vi "DualEncoder.vi"(8 "error in (no error)":errorcluster, 11 "Reset?":bool) -> (0 "error out":errorcluster, 1 "Distance Right (in)":dbl, 2 "Distance Left (in)":dbl, 3 "Total Distance (in)":dbl, 4 "Angle (degrees)":dbl)   [LabVIEW 2012]
uses:
  Robot Global Data.vi
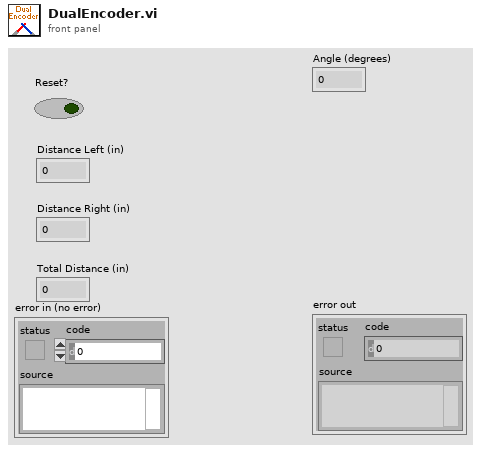
[diagram p1: front panel]
types:
  T1 = typedef "WPI_EncoderDevRef.ctl" = cluster{"DevStatus":errorcluster, "EncoderIndex":T2, "CounterIndex":T3, "DistancePerCount":dbl, "Decoding Type":T4}
  T2 = typedef "FPGA_EncoderIdx.ctl" = enum8{"Enc 0", "Enc 1", "Enc 2", "Enc 3", "Invalid"}
  T3 = typedef "FPGA_CounterCtrSystemIndex.ctl" = enum8{"Ctr 0", "Ctr 1", "Ctr 2", "Ctr 3", "Ctr 4", "Ctr 5", "Ctr 6", "Ctr 7", "Invalid"}
  T4 = typedef "WPI_EncoderType.ctl" = enum16{"1x", "2x", "4x"}
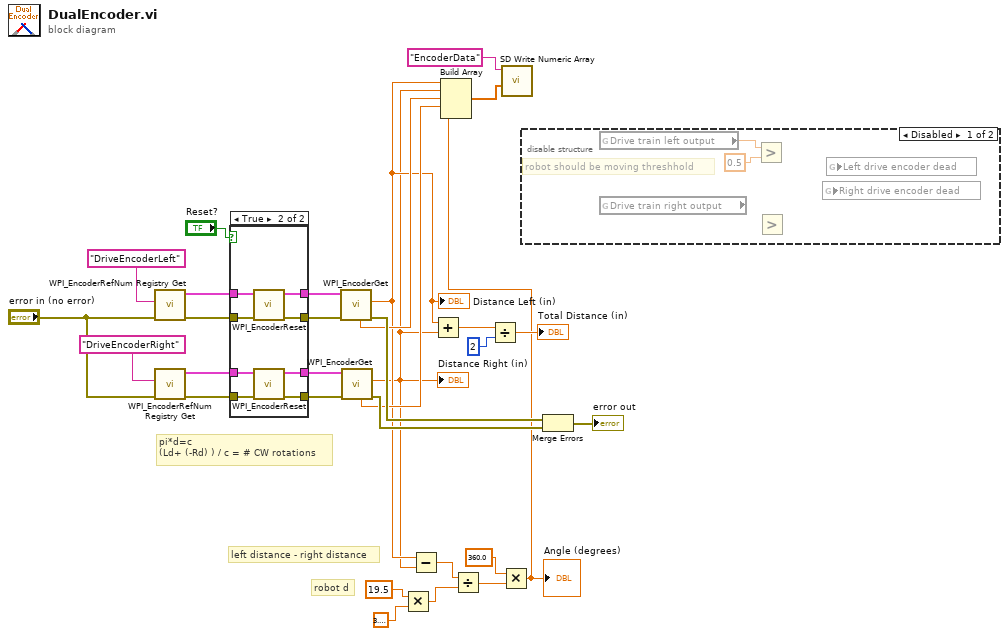
[diagram p0: block diagram]
diagram:
  # "left distance - right distance"
  # "robot d"
  # "pi*d=c\n(Ld+ (-Rd) ) / c = # CW rotations"
  n1 = call <vilib>:"WPI_EncoderRefNum Registry Get.vi"("error in (no error)"="error in (no error)", "refnum name"="DriveEncoderLeft") -> ("error out"=w25:errorcluster, "EncoderDevRef"=w26:T1)  [unwired: 8 in]
  n2 = call <vilib>:"WPI_EncoderRefNum Registry Get.vi"("error in (no error)"="error in (no error)", "refnum name"="DriveEncoderRight") -> ("error out"=w27:errorcluster, "EncoderDevRef"=w28:T1)  [unwired: 8 in]
  n3 = case shown="True" "Reset?" {
    tunnel: w28 -> [w33 w43]
    tunnel: w27 -> [w32 w42]
    tunnel: w26 -> [w35 w41]
    tunnel: w25 -> [w34 w40]
    tunnel: [w35 w39] -> w23
    tunnel: [w34 w38] -> w22
    tunnel: [w33 w37] -> w21
    tunnel: [w32 w36] -> w20
    frame False {
    }
    frame True {
      n4 = call <vilib>:"WPI_EncoderReset.vi"("error in (no error)"=w40, "EncoderDevRef"=w41) -> ("error out"=w38:errorcluster, "EncoderDevRef"=w39:T1)  [unwired: 8 in]
      n5 = call <vilib>:"WPI_EncoderReset.vi"("error in (no error)"=w42, "EncoderDevRef"=w43) -> ("error out"=w36:errorcluster, "EncoderDevRef"=w37:T1)  [unwired: 8 in]
    }
  }
  n6 = call <vilib>:"WPI_EncoderGet.vi"("error in (no error)"=w22, "EncoderDevRef"=w23) -> ("error out"=w16:errorcluster, "Distance"=w9:dbl, "Rate"=w11:dbl)  [unwired: 4 in, 3 out]
  "Distance Left (in)" <- w9
  n7 = call <vilib>:"WPI_EncoderGet.vi"("error in (no error)"=w20, "EncoderDevRef"=w21) -> ("error out"=w15:errorcluster, "Distance"=w8:dbl, "Rate"=w10:dbl)  [unwired: 4 in, 3 out]
  "Distance Right (in)" <- w8
  n8 = Multiply(x=19.5, y=3.141592653589793) -> (x*y=w4:dbl)
  n9 = Subtract(x=w9, y=w8) -> (x-y=w5:dbl)
  n10 = Add(x=w9, y=w8) -> (x+y=w18:dbl)
  n11 = Divide(x=w5, y=w4) -> (x/y=w3:dbl)
  n12 = Divide(x=w18, y=2) -> (x/y=→"Total Distance (in)":dbl)
  n13 = Multiply(x=360.0, y=w3) -> (x*y=w1:dbl)
  "Angle (degrees)" <- w1
  n14 = Build Array(w9, w8, w11, w10, w1) -> (w12:dbl[])
  n15 = call <vilib>:"SD Write Numeric Array.vi"("Numeric Array"=w12, "Name"="EncoderData") -> ()  [unwired: 8 in, 2 out]
  n16 = disable-structure shown="Disabled" {
    frame Disabled {
      # "robot should be moving threshhold"
      n17 = global read "Robot Global Data.vi" "Drive train left output"() -> (w45:dbl)
      n18 = global read "Robot Global Data.vi" "Drive train right output"() -> ()  [unwired: 1 out]
      n19 = Greater?(x=w45, y=0.5) -> ()  [unwired: 1 out]
      n20 = Greater?() -> ()  [unwired: 2 in, 1 out]
      n21 = global read "Robot Global Data.vi" "Right drive encoder dead"() -> ()  [unwired: 1 in]
      n22 = global read "Robot Global Data.vi" "Left drive encoder dead"() -> ()  [unwired: 1 in]
    }
    frame Enabled {
    }
  }
  n23 = Merge Errors(w16, w15) -> (→"error out":errorcluster)
